vi "IDE_msg_Example.vi"() -> ()   [LabVIEW 2020]
uses:
  Subs/ColorText/Code.xctl
  Subs/Console XCtrl/Console_Xctrl.xctl
  Subs/Server XCtrl/Server.xctl
  Subs/SystemLink/SL_Subs/SL_XControl.xctl
  Subs/SystemLink/SL_Subs/SystemLink_Write_String.vi
panel:
  in  "SystemLink":string(xcontrol)="fred"
  in  "Clean":bool
  in  "PC Save":bool
  in  "PC path":path
  in  "Files":bool
  in  "Server":bool
  in  "Help":bool
  in  "Server":path(xcontrol)=path "/Users/crogers/GitHub/Summer2020/LabVIEWCode/Servers/Jens.vi"
  out "REPL":string(xcontrol)="\n>>> import hub,utime\n>>> ser = hub.USB_VCP()\n>>> \n>>> mbegin=b'msg_start\\n'\n>>> mend=b'\\nmsg_end\\n'\n>>> rbegin = b'reply_start'\n>>> rend = b'reply_end'\n>>> \n>>> def comm(payload):\n...     s =  b' '\n...     ser.write(mbegin + payload + mend)\n...     utime.sleep(0.01)\n...     while not(rend in s):\n...         try:\n...             s = s + ser.readline()\n...             #print(s) \n...         except:\n...             utime.sleep(0.1)\n...     start = len(rbegin)+s.find(rbegin)\n...     end = s.find(rend)\n...     reply = s[start:end]\n...     utime.sleep(1)\n...     return reply.decode()\n... \n>>> \n>>> reply = comm(b\"send to pc\")\nmsg_start\nsend to pc\nmsg_end\n>>> reply_start send to pc reply_endreply_start send to pc reply_endreply_start send to pc reply_end"
  in  "Clear":bool
  in  "Save":bool
  in  "Stop":bool
  in  "Run":bool
  in  "Name":string="code.py"
  in  "Code":string(xcontrol)="import hub,utime\r\nser = hub.USB_VCP()\r\n\r\nmbegin=b'msg_start\\n'\r\nmend=b'\\nmsg_end\\n'\r\nrbegin = b'reply_start '\r\nrend = b' reply_end'\r\n\r\ndef comm(payload):\r\n    s =  b' '\r\n    ser.write(mbegin + payload + mend)\r\n    utime.sleep(0.01)\r\n    while not(rend in s):\r\n        try:\r\n            s = s + ser.readline()\r\n            print(s)  \r\n        except:\r\n            utime.sleep(0.1)\r\n    start = len(rbegin)+s.find(rbegin)\r\n    end = s.find(rend)\r\n    reply = s[start:end]\r\n    return reply.decode()\r\n\r\nreply = [b'']*10   \r\nfor i in range(10):\r\n    reply[i] = comm(b\"send to pc \" + str(i))\r\n    print(reply[i])\r"
  # "¨Processor"
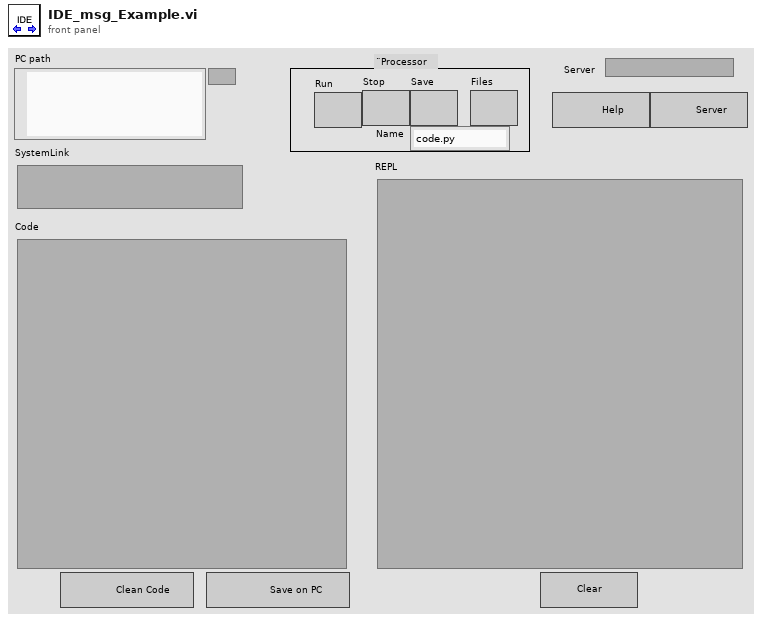
[diagram p1: front panel]
types:
  T1 = cluster{"Quote":u32, "Comment":u32, "Python":u32, "Text":u32, "Triple Quote":u32, "function":u32, "Line numbers":u32, "REPL Err":u32, "REPL Text":u32, "Text Bkgd":u32, "REPL Bkgd":u32}
  T2 = enum8{"Enabled", "Disabled", "Disabled and Grayed Out"}
  T3 = typedef "eventvkey.ctl" = enum16{"ASCII", "Enter", "Return", "Shift", "Ctrl", "Alt", "Cmd", "Opt", "Caps", "NumLock", "Clear", "Break", "Up", "Down", "Left", "Right", "Insert", "Delete", "Home", "End", "PageUp", "PageDown", "Escape", "Help", "Pause", "ScrollLock", "F1", "F2", "F3", "F4", "F5", "F6", "F7", "F8", "F9", "F10", "F11", "F12", "F13", "F14", "F15", "F16", "F17", "F18", "F19", "F20", "F21", "F22", "F23", "F24", "Play", "VolumeUp", "VolumeDown", "Mute", "Two Byte Char"}
  T4 = cluster{"Shift":bool, "Ctrl":bool, "Alt":bool, "Cmd":bool, "Opt":bool}
  T5 = cluster{"Char":i16, "VKey":T3, "PlatMods":cluster{"Shift":bool, "Ctrl":bool, "Alt":bool, "Cmd":bool, "Opt":bool}}
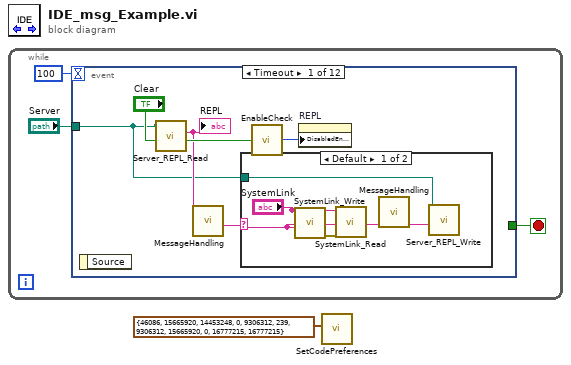
[diagram p0: block diagram]
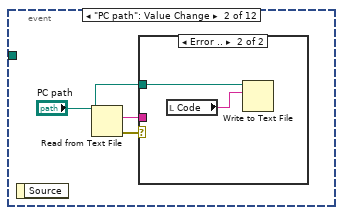
[diagram p3: hidden frame]
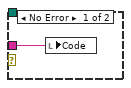
[diagram p4: hidden frame]
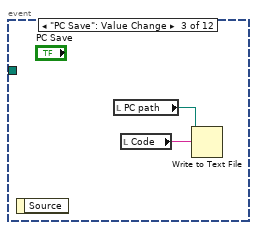
[diagram p5: hidden frame]
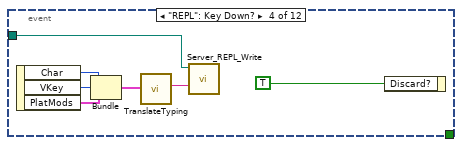
[diagram p6: hidden frame]
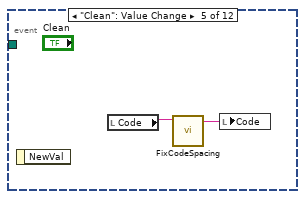
[diagram p7: hidden frame]
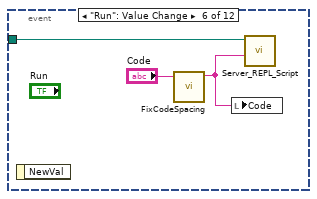
[diagram p8: hidden frame]
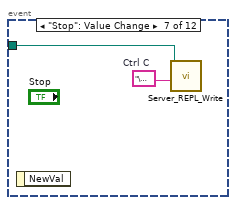
[diagram p9: hidden frame]
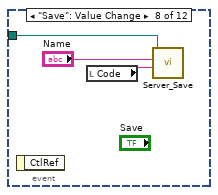
[diagram p10: hidden frame]
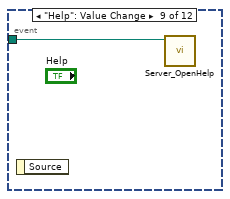
[diagram p11: hidden frame]
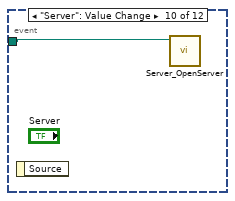
[diagram p12: hidden frame]
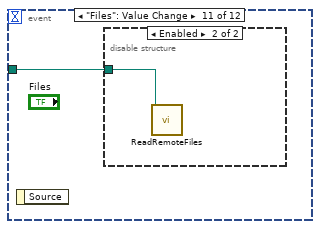
[diagram p13: hidden frame]
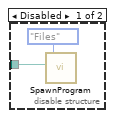
[diagram p14: hidden frame]
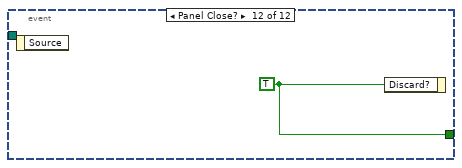
[diagram p15: hidden frame]
diagram:
  n1 = while {
    stop <- w3 stop-if-true
    n2 = event shown="[0] Timeout" {
      selector: _ -> [_ _ _ _ _ _ _ _ _ _ _ _]
      dyn-events: _ -> [_ _ _ _ _ _ _ _ _ _ _ _]
      timeout: 100 -> [_ _ _ _ _ _ _ _ _ _ _ _]
      tunnel: [_ _ _ _ _ _ _ _ _ _ _ w47] -> w3
      tunnel: "Server" -> [w5 _ _ w24 _ w34 w36 w38 w41 w42 w43 _]
      event Timeout {
        n3 = event-data() -> ()  [unwired: 1 in, 1 out]
        n4 = call "Server_REPL_Read.vi"("Clear"="Clear", "Server"=w5) -> ("Running?"=w9:bool, "REPL"=w7:string)  [unwired: 7 in, 1 out]
        "REPL" <- w7
        n5 = call "MessageHandling.vi"("REPL"=w7) -> ("New Message"=w6:string)  [unwired: 7 in, 3 out]
        n6 = case shown="Default" w6 {
          selector: w6 -> [w11 _]
          tunnel: w5 -> [w13 _]
          frame Default {
            n7 = call-poly "SystemLink_Write.vi"("String"=w11, "SL_XControl"="SystemLink") -> ("error out"=w15:errorcluster)  [unwired: 9 in]
            n8 = call "SystemLink_Read.vi"("error in"=w15, "SystemLink Tag"="SystemLink") -> ()  [unwired: 6 in, 4 out]
            n9 = call "MessageHandling.vi"("Reply"=w11) -> ("New Reply"=w12:string)  [unwired: 7 in, 3 out]
            n10 = call "Server_REPL_Write.vi"("Code"=w12, "Server"=w13) -> ()  [unwired: 9 in, 1 out]
          }
          frame "" {
          }
        }
        n11 = call "EnableCheck.vi"("Enable?"=w9) -> ("Enum"=w10:T2)
        n12 = property on="REPL" class="Console_Xctrl (strict)"("DisabledEnum"=w10) -> ()  [unwired: 2 in, 2 out]
      }
      event "PC path": Value Change {
        n13 = event-data() -> ()  [unwired: 1 in, 1 out]
        n14 = Read from Text File(file (use dialog)="PC path") -> (text=w17:string, error out=w18:errorcluster)  [unwired: 3 in, 2 out]
        n15 = case shown="Error .." w18 {
          tunnel: w17 -> [w19 _]
          tunnel: "PC path" -> [_ w21]
          frame No Error {
            n16 = local write "Code"(w19) -> ()
          }
          frame Error {
            n17 = local read "Code"() -> (w20:string)
            n18 = Write to Text File(file (use dialog)=w21, text=w20) -> ()  [unwired: 2 in, 3 out]
          }
        }
      }
      event "PC Save": Value Change {
        n19 = event-data() -> ()  [unwired: 1 in, 1 out]
        n20 = local read "PC path"() -> (w23:path)
        n21 = local read "Code"() -> (w22:string)
        n22 = Write to Text File(file (use dialog)=w23, text=w22) -> ()  [unwired: 2 in, 3 out]
      }
      event "REPL": Key Down? {
        n23 = event-data() -> ("Char"=w29:i16, "VKey"=w28:T3, "PlatMods"=w26:T4)  [unwired: 1 in]
        n24 = Bundle("Char"=w29, "VKey"=w28, "PlatMods"=w26) -> (w30:T5)  [unwired: 1 in]
        n25 = call "TranslateTyping.vi"("Cluster"=w30) -> ("key"=w25:string)  [unwired: 10 in]
        n26 = call "Server_REPL_Write.vi"("Code"=w25, "Server"=w24) -> ()  [unwired: 9 in, 1 out]
        n27 = event-data("Discard?"=TRUE) -> ()  [unwired: 1 in, 1 out]
      }
      event "Clean": Value Change {
        n28 = event-data() -> ()  [unwired: 1 in, 1 out]
        n29 = local read "Code"() -> (w31:string)
        n30 = call "FixCodeSpacing.vi"("Code"=w31) -> ("Cleaned"=w32:string)  [unwired: 10 in]
        n31 = local write "Code"(w32) -> ()
      }
      event "Run": Value Change {
        n32 = event-data() -> ()  [unwired: 1 in, 1 out]
        n33 = call "FixCodeSpacing.vi"("Code"="Code") -> ("Cleaned"=w33:string)  [unwired: 10 in]
        n34 = local write "Code"(w33) -> ()
        n35 = call "Server_REPL_Script.vi"("Code"=w33, "Server"=w34) -> ()  [unwired: 9 in, 1 out]
      }
      event "Stop": Value Change {
        w37 = "\u0003"  # Ctrl C
        n36 = event-data() -> ()  [unwired: 1 in, 1 out]
        n37 = call "Server_REPL_Write.vi"("Code"=w37, "Server"=w36) -> ()  [unwired: 9 in, 1 out]
      }
      event "Save": Value Change {
        n38 = event-data() -> ()  [unwired: 1 in, 1 out]
        n39 = local read "Code"() -> (w40:string)
        n40 = call "Server_Save.vi"("Code"=w40, "Name"="Name", "Server"=w38) -> ()  [unwired: 8 in, 1 out]
      }
      event "Help": Value Change {
        n41 = event-data() -> ()  [unwired: 1 in, 1 out]
        n42 = call "Server_OpenHelp.vi"("Server"=w41) -> ()  [unwired: 10 in, 1 out]
      }
      event "Server": Value Change {
        n43 = event-data() -> ()  [unwired: 1 in, 1 out]
        n44 = call "Server_OpenServer.vi"("Server"=w42) -> ()  [unwired: 10 in, 1 out]
      }
      event "Files": Value Change {
        n45 = event-data() -> ()  [unwired: 1 in, 1 out]
        n46 = disable-structure shown="Enabled" {
          disable-tunnel: w43 -> [w44 w46]
          frame Disabled {
            n47 = call "SpawnProgram.vi"("Server"=w44, "Dialog"=enum16{"Help", "Files"}."Files") -> ()  [unwired: 10 in]
          }
          frame Enabled {
            n48 = call "ReadRemoteFiles.vi"("Server"=w46) -> ()  [unwired: 11 in]
          }
        }
      }
      event Panel Close? {
        w47 = TRUE ("Discard?")
        n49 = event-data() -> ()  [unwired: 1 in, 1 out]
        n50 = event-data("Discard?"=w47) -> ()  [unwired: 1 in, 1 out]
      }
    }
  }
  n51 = call "SetCodePreferences.vi"("Color choices"=T1 {"Quote"=46086, "Comment"=15665920, "Python"=14453248, "Text"=0, "Triple Quote"=9306312, "function"=239, "Line numbers"=9306312, "REPL Err"=15665920, "REPL Text"=0, "Text Bkgd"=16777215, "REPL Bkgd"=16777215}) -> ()  [unwired: 11 in]
